vi "Lookup Descendants.vi"(8 "error in (no error)":errorcluster, 10 "Lookup":refnum<class "Config Lookup.lvclass">, 11 "Config Element in":refnum<class "Config Element.lvclass">) -> (0 "error out":errorcluster, 2 "Descendants":refnum<class "Config Element.lvclass">[](array[class]), 3 "Config Element out":refnum<class "Config Element.lvclass">)   [LabVIEW 2020, in "CDM-Config.lvlib" / "Config Element.lvclass"]
uses:
  Config Element.lvclass
  Config Element.lvclass/Config Element.ctl
  Config Manager/Config Manager.lvclass
  Config Filter/Config Lookup.lvclass
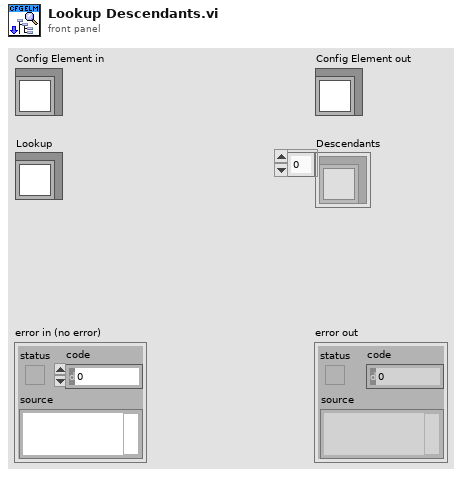
[diagram p1: front panel]
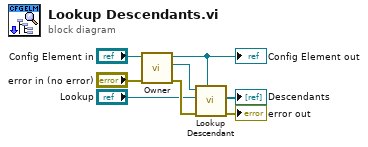
[diagram p0: block diagram]
diagram:
  n1 = call "Owner.vi"("error in (no error)"="error in (no error)", "Config Element in"="Config Element in") -> ("error out"=w8:errorcluster, "Owner"=w5:refnum<class "Config Manager.lvclass">, "Config Element out"=w4:refnum<class "Config Element.lvclass">)  [unwired: 7 in]
  "Config Element out" <- w4
  n2 = call "Lookup Descendant.vi"("Start (Root)"=w4, "error in (no error)"=w8, "Lookup"="Lookup", "Config Manager in"=w5) -> ("error out"=→"error out":errorcluster, "Descendants"=→"Descendants":refnum<class "Config Element.lvclass">[])  [unwired: 5 in, 1 out]
